vi "ClearFaults.vi"(11 "DA in":refnum<class "DA.lvclass">) -> (3 "DA out":refnum<class "DA.lvclass">)   [LabVIEW 2019, in "DA.lvclass"]
uses:
  DA.lvclass
  DA.lvclass/DA.ctl
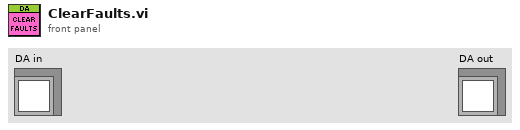
[diagram p1: front panel]
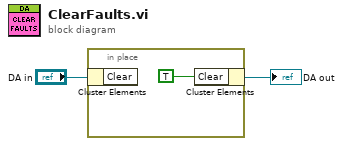
[diagram p0: block diagram]
diagram:
  n1 = in-place {
    n2 = in-place-cluster #1("DA in") -> ()  [unwired: 1 out]
    n3 = in-place-cluster #1("Clear"=TRUE ("bool_data.CURR")) -> (→"DA out":refnum<class "DA.lvclass">)
  }
